vi "Init.vi"(8 "error in":errorcluster, 11 "Image in":refnum<class "Image.lvclass">) -> (0 "error out":errorcluster, 3 "Image out":refnum<class "Image.lvclass">)   [LabVIEW 2023, in "SourceGrid.lvlib" / "Image.lvclass"]
uses:
  Image.lvclass
  D:/git/Sourcegrid-LabVIEW/dll/SourceGrid.dll
  dll/SourceGrid.dll
  Cell/Cell.lvclass
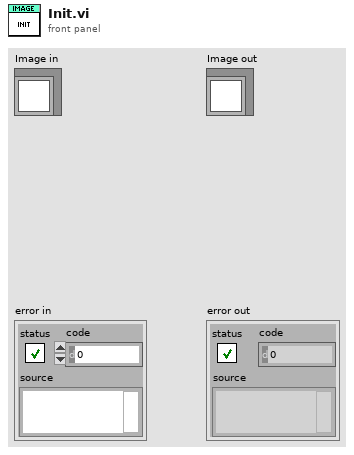
[diagram p1: front panel]
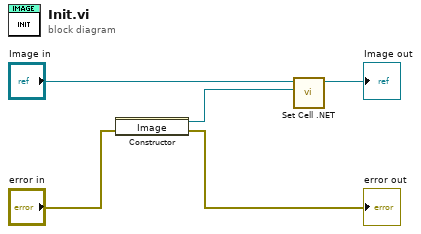
[diagram p0: block diagram]
diagram:
  n1 = constructor class="Image"(error in="error in") -> (reference out=w1:refnum<k24>, error out=→"error out":errorcluster)  [unwired: 2 in, 1 out]
  n2 = call "Set Cell .NET.vi"("Cell .NET"=w1, "Cell in"="Image in") -> ("Cell out"=→"Image out":refnum<class "Image.lvclass">)  [unwired: 9 in]
